vi "Port Open.vi"(8 "error in (no error)":errorcluster, 11 "SJ-210 in":refnum<class "SJ-210.lvclass">) -> (0 "error out":errorcluster, 3 "SJ-210 out":refnum<class "SJ-210.lvclass">)   [LabVIEW 2014, in "SJ-210.lvlib" / "SJ-210.lvclass"]
doc: "Abre el puerto COM que indica el usuario y setea valores por defecto al puerto."
uses:
  SJ-210.lvclass
  SJ-210.lvclass/SJ-210.ctl
  API/SJ-210 Lib.lvlib
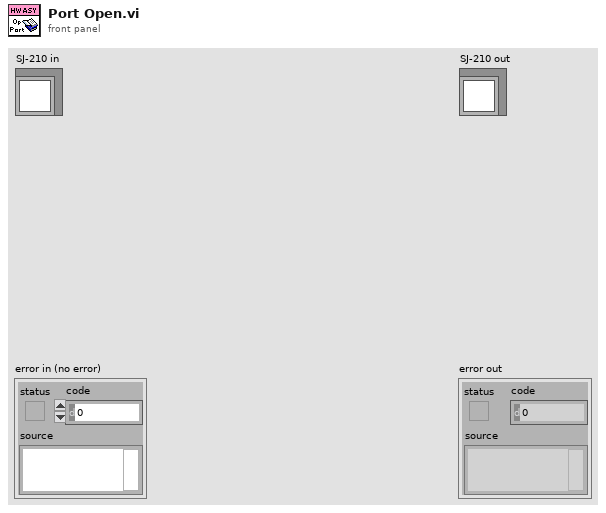
[diagram p1: front panel]
types:
  T1 = cluster{"VISA resource name":refnum<visa-resource-name>}
  T2 = typedef "SJ-210 Lib.lvlib/Connection Data.ctl" = cluster{"VISA resource name":refnum<visa-resource-name>}
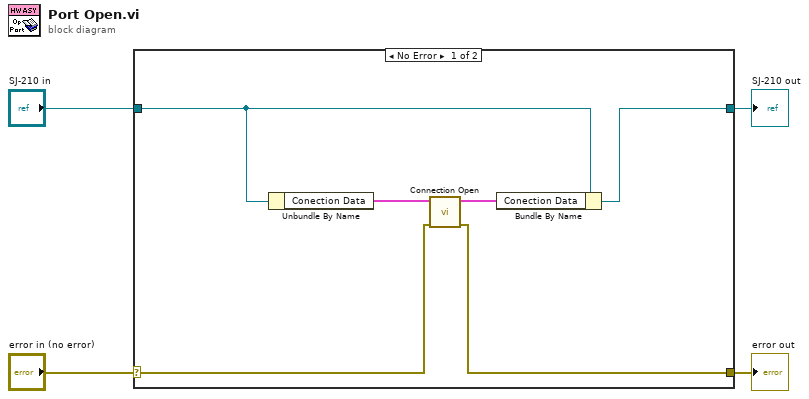
[diagram p0: block diagram]
diagram:
  n1 = case shown="No Error" "error in (no error)" {
    selector: "error in (no error)" -> [w6 w12]
    tunnel: [w5 w12] -> w3
    tunnel: [w7 w11] -> w1
    tunnel: "SJ-210 in" -> [w8 w11]
    frame No Error {
      n2 = Unbundle By Name(w8) -> ("Conection Data"=w10:T1)
      n3 = call "Connection Open.vi"("error in (no error)"=w6, "Conection Data"=w10) -> ("error out"=w5:errorcluster, "Conection Data Out"=w9:T2)  [unwired: 8 in]
      n4 = Bundle By Name(cluster=w8, "Conection Data"=w9) -> (w7:refnum<class "SJ-210.lvclass">)
    }
    frame Error {
    }
  }
  "error out" <- w3
  "SJ-210 out" <- w1
